vi "FPGA_bubble_loop.vi"() -> ()   [LabVIEW 2020]
uses:
  <vilib>/rvi/Emulation/niFpgaGetClockAttributes.vi
  <vilib>/rvi/Emulation/niFpgaSctlEmulationGetInTimedLoop.vi
  <vilib>/rvi/Emulation/niFpgaEmulationReportErrorSimple.vi
  <vilib>/rvi/Emulation/niFpgaCriticalErrorInLSC.vi
  <vilib>/rvi/DataTransferAndStorage/Container/XNode/niFpgaContainer.xnode
  <vilib>/rvi/interface/RandomDataEmulation/nirviRandomDataFpgaReadWriteTemplate.vi
  <vilib>/rvi/FIFO/Fifo_Resource/nirvififoEmulationWrite.vi
panel:
  out "index Array":i32[](array[numeric])
  out "Output Valid":bool
  out "Sorted array":u8[](array[numeric])
  out "Sorted index":u8[](array[numeric])
  in  "Input Array":u8[](array[numeric])=[0, 0, 0, 0, 0, 0, 0, 0]
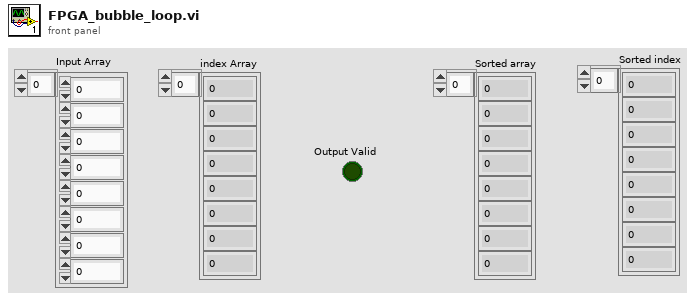
[diagram p1: front panel]
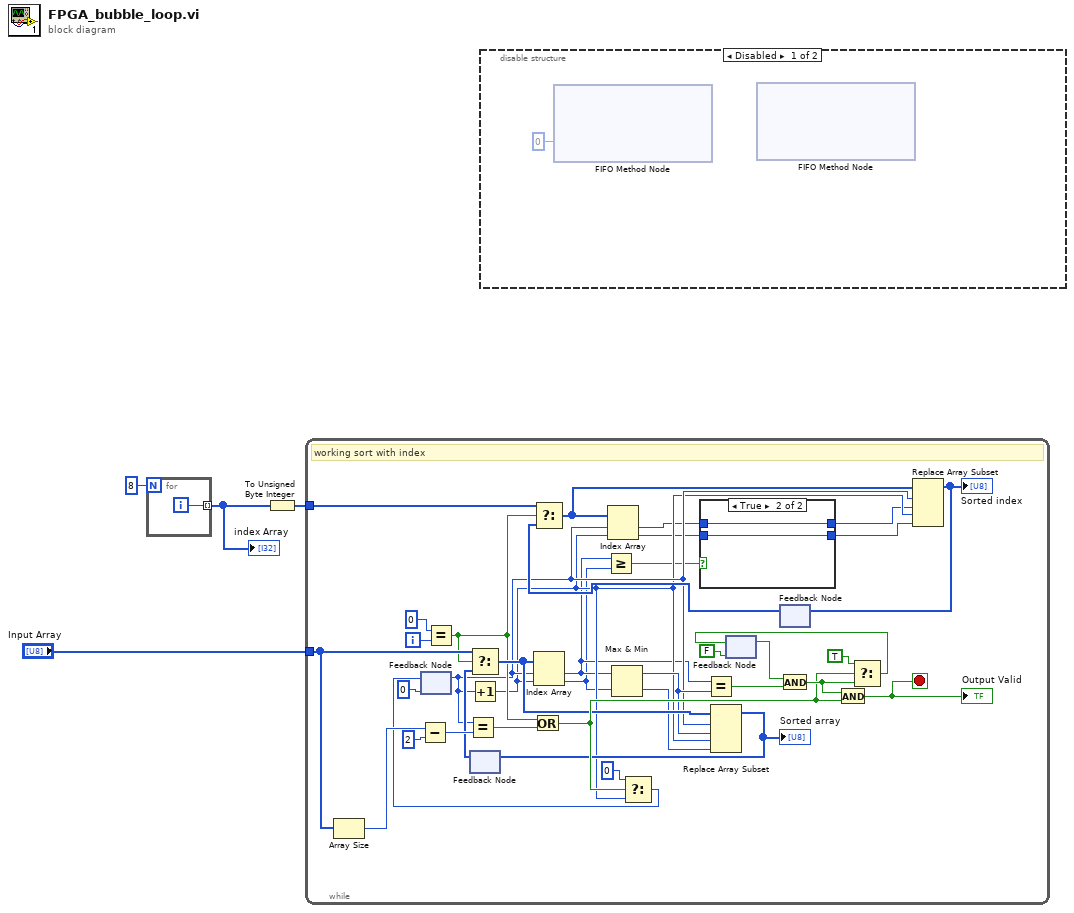
[diagram p0: block diagram]
diagram:
  n1 = for {
    N: 8 -> [_]
    tunnel: [w5] -> w3 mode=indexing
    i -> [w5]
  }
  "index Array" <- w3
  n2 = To Unsigned Byte Integer(number=w3) -> (unsigned 8bit integer=w2:u8[])
  n3 = while {
    tunnel: "Input Array" -> [w39]
    tunnel: w2 -> [w17]
    i -> [w21]
    stop <- w22 stop-if-true
    # "working sort with index"
    n4 = Array Size(array=w39) -> (size(s)=w42:i32)
    n5 = Subtract(x=w42, y=2) -> (x-y=w40:i32)
    n6 = feedback #1(0 ("y")) -> (w15:i32)
    n7 = Equal?(x=0, y=w21) -> (x = y?=w16:bool)
    n8 = Equal?(x=w15, y=w40) -> (x = y?=w27:bool)
    n9 = Increment(x=w15) -> (x+1=w14:i32)
    n10 = feedback #2() -> (w32:u8[])  [unwired: 1 in]
    n11 = Select(t=w39, s=w16, f=w32) -> (s? t:f=w26:u8[])
    n12 = Or(x=w16, y=w27) -> (x .or. y?=w30:bool)
    n13 = Index Array(array=w26, index #1=w15, index #2=w14) -> (element #1=w8:u8, element #2=w7:u8)
    n14 = Greater Or Equal?(x=w8, y=w7) -> (x >= y?=w6:bool)
    n15 = Max & Min(x=w8, y=w7) -> (max(x,y)=w24:u8, min(x,y)=w23:u8)
    n16 = Select(t=0 ("y"), s=w30, f=w14) -> (s? t:f=w28:i32)
    n17 = feedback-in #1(w28) -> ()
    n18 = Equal?(x=w8, y=w24) -> (x = y?=w38:bool)
    n19 = Replace Array Subset(array=w26, new element #1=w24, index #1=w15, new element #2=w23, index #2=w14) -> (w25:u8[])
    "Sorted array" <- w25
    n20 = feedback-in #2(w25) -> ()
    n21 = feedback #3(FALSE ("t")) -> (w35:bool)
    n22 = feedback #4() -> (w19:u8[])  [unwired: 1 in]
    n23 = Select(t=w17, s=w16, f=w19) -> (s? t:f=w18:u8[])
    n24 = Index Array(array=w18, index #1=w15, index #2=w14) -> (element #1=w12:u8, element #2=w9:u8)
    n25 = case shown="True" w6 {
      tunnel: w12 -> [w44 w46]
      tunnel: [w43 w46] -> w11
      tunnel: [w44 w45] -> w10
      tunnel: w9 -> [w43 w45]
      frame False {
      }
      frame True {
      }
    }
    n26 = And(x=w35, y=w38) -> (x .and. y?=w33:bool)
    n27 = And(x=w33, y=w30) -> (x .and. y?=w22:bool)
    "Output Valid" <- w22
    n28 = Select(t=TRUE, s=w30, f=w33) -> (s? t:f=w36:bool)
    n29 = feedback-in #3(w36) -> ()
    n30 = Replace Array Subset(array=w18, new element #1=w11, index #1=w15, new element #2=w10, index #2=w14) -> (w13:u8[])
    "Sorted index" <- w13
    n31 = feedback-in #4(w13) -> ()
  }
  n32 = disable-structure shown="Disabled" {
    frame Disabled {
      n33 = xnode ("FIFO Method Node")("Timeout"=0) -> ()  [unwired: 1 in, 3 out]
      n34 = xnode ("FIFO Method Node")() -> ()  [unwired: 3 in, 2 out]
    }
    frame Enabled {
    }
  }
